vi "Sequence Basicdata inquiry.vi"(7 "Channel  (1: CH1)":u16(ring)=1 items=["CH1"=1, "CH2"=2, "CH3"=3, "CH4"=4], 8 "error in (no error)":errorcluster, 11 "VISA resource name":refnum<visa-resource-name>) -> (0 "error out":errorcluster, 1 "Start":string, 2 "Cycles":string, 3 "VISA resource name out":refnum<visa-resource-name>, 4 "End State":string, 6 "Groups":string)   [LabVIEW 2020, in "GPP.lvlib"]
uses:
  GPP.lvlib
  Function/VISA_COMMON.ctl
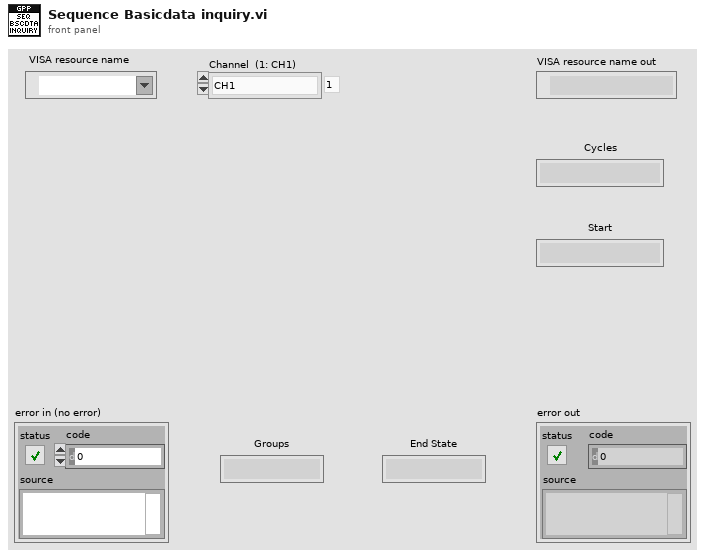
[diagram p1: front panel]
types:
  T1 = typedef "GPP.lvlib/VISA_COMMON.ctl" = enum16{"Initial", "Write CMD", "Read Result", "Read History", "Close"}
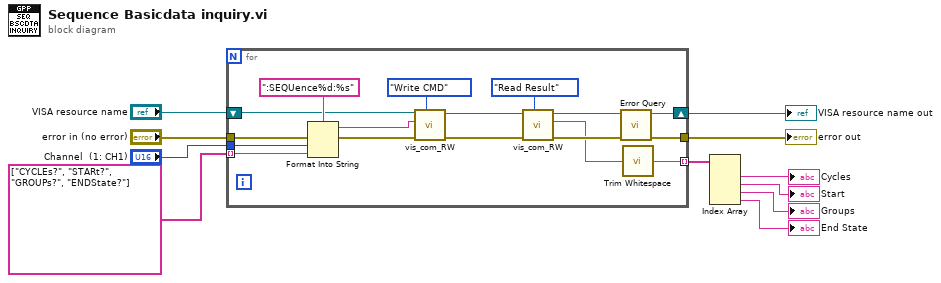
[diagram p0: block diagram]
diagram:
  n1 = for {
    tunnel: "error in (no error)" -> [w22]
    tunnel: "Channel  (1: CH1)" -> [w20]
    tunnel: string[] ["CYCLEs?", "STARt?", "GROUPs?", "ENDState?"] -> [w17] mode=indexing
    tunnel: [w18] -> w6
    tunnel: [w14] -> w8 mode=indexing
    shift-right: [w12] -> w5
    shift-left: "VISA resource name" -> [w16]
    n2 = Format Into String(format string=":SEQUence%d:%s", error in=w22, w20, w17) -> (resulting string=w15:string, error out=w21:errorcluster)  [unwired: 1 in]
    n3 = call "vis_com_RW.vi"("Funciton"=VISA_COMMON."Write CMD", "error in (no error)"=w21, "CMD String"=w15, "VISA resource in"=w16) -> ("error out"=w26:errorcluster, "VISA resource out"=w25:refnum<visa-resource-name>)  [unwired: 5 in, 1 out]
    n4 = call "vis_com_RW.vi"("Funciton"=VISA_COMMON."Read Result", "error in (no error)"=w26, "VISA resource in"=w25) -> ("error out"=w23:errorcluster, "Result"=w13:string, "VISA resource out"=w24:refnum<visa-resource-name>)  [unwired: 6 in]
    n5 = call "Error Query.vi"("error in (no error)"=w23, "VISA resource name"=w24) -> ("error out"=w18:errorcluster, "VISA resource name out"=w12:refnum<visa-resource-name>)  [unwired: 6 in, 2 out]
    n6 = call <vilib>:"Trim Whitespace.vi"("string"=w13) -> ("trimmed string"=w14:string)  [unwired: 1 in]
  }
  "error out" <- w6
  "VISA resource name out" <- w5
  n7 = Index Array(array=w8) -> (element #1=→"Cycles":string, element #2=→"Start":string, element #3=→"Groups":string, element #4=→"End State":string)  [unwired: 4 in]
